vi "2.1.vi"(1 "b":dbl, 2 "x":dbl, 3 "k":dbl) -> (0 "y":dbl)   [LabVIEW 2017]
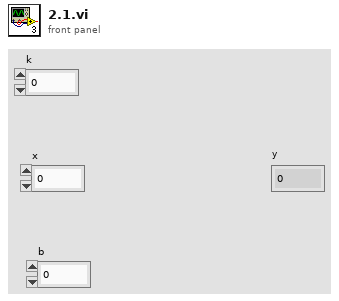
[diagram p1: front panel]
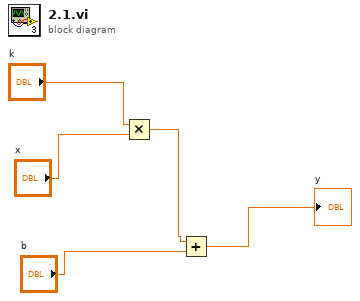
[diagram p0: block diagram]
diagram:
  n1 = Multiply(x="k", y="x") -> (x*y=w3:dbl)
  n2 = Add(x=w3, y="b") -> (x+y=→"y":dbl)
